vi "niP2P Unlink Peer to Peer Stream.vi"(0 "stream session":refnum<k20>, 11 "error in (no error)":errorcluster) -> (4 "stream session out":refnum<k20>, 15 "error out":errorcluster)   [LabVIEW 2010]
doc: "Unlinks the reader and writer in the stream you specify. If the stream is enabled, this VI disables the stream before unlinking the reader and writer."
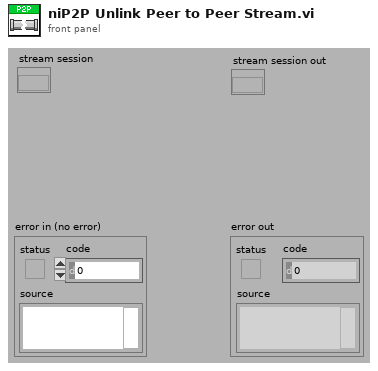
[diagram p1: front panel]
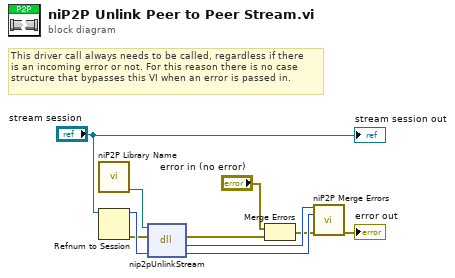
[diagram p0: block diagram]
diagram:
  # "This driver call always needs to be called, regardless if there\nis an incoming error or not. For this reason there is no case\nstructure that bypasses this VI when an error is passed in."
  n1 = call <vilib>:"niP2P Library Name.vi"() -> ("nip2p libname"=w3:path)  [unwired: 10 in]
  n2 = Refnum to Session(7:"stream session") -> (0:w2:errorcluster, 3:w9:u64)  [unwired: 1 in]
  n3 = dll-call lib="?" fn="nip2pUnlinkStream"(path in=w3, error in=w2, "streamHandle"=w9) -> (error out=w1:errorcluster, "return type"=w7:i32, "streamHandle"=w6:u32)  [unwired: 1 in, 1 out]
  n4 = Merge Errors("error in (no error)", w1) -> (w5:errorcluster)
  n5 = call <vilib>:"niP2P Merge Errors.vi"("error code"=w7, "stream handle (0)"=w6, "error in"=w5) -> ("error out"=→"error out":errorcluster)  [unwired: 12 in]
  "stream session out" <- "stream session"
